vi "Remove datafiles from data folder (subVi).vi"(1 "error in":errorcluster) -> (0 "error out":errorcluster)   [LabVIEW 2016]
uses:
  global/Config_Infos.vi
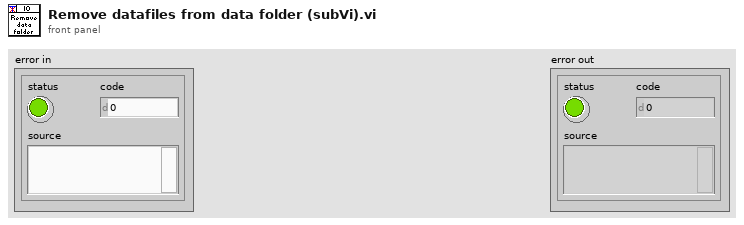
[diagram p1: front panel]
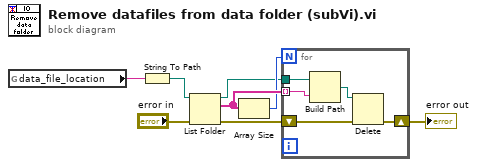
[diagram p0: block diagram]
diagram:
  n1 = global read "Config_Infos.vi" "data_file_location"() -> (w8:string)
  n2 = String To Path(string=w8) -> (path=w7:path)
  n3 = List Folder(path=w7, error in="error in") -> (path out=w4:path, filenames=w6:string[], error out=w3:errorcluster)  [unwired: 2 in, 1 out]
  n4 = Array Size(array=w6) -> (size(s)=w5:i32)
  n5 = for {
    N: w5 -> [_]
    tunnel: w6 -> [w12] mode=indexing
    tunnel: w4 -> [w13]
    shift-right: [w11] -> w1
    shift-left: w3 -> [w9]
    n6 = Build Path(base path=w13, name or relative path=w12) -> (appended path=w10:path)
    n7 = Delete(path (use dialog)=w10, error in=w9) -> (error out=w11:errorcluster)  [unwired: 3 in, 2 out]
  }
  "error out" <- w1
